vi "GetTaskInfo.vi"(0 "error in":errorcluster, 5 "Telnet":refnum<k24>, 9 "task":string) -> (4 "error out":errorcluster, 6 "KclCommand":string, 8 "Succeed":bool, 10 "ErrorText":string, 15 "TaskInfo":T1)   [LabVIEW 2024, in "UnderAutomation.Fanuc.lvlib"]
uses:
  UnderAutomation.Fanuc.lvlib
  C:/Users/fg/Documents/Fanuc.vi/LabVIEW_2024/UnderAutomation.Fanuc/lib/UnderAutomation.Fanuc.dll
  lib/UnderAutomation.Fanuc.dll
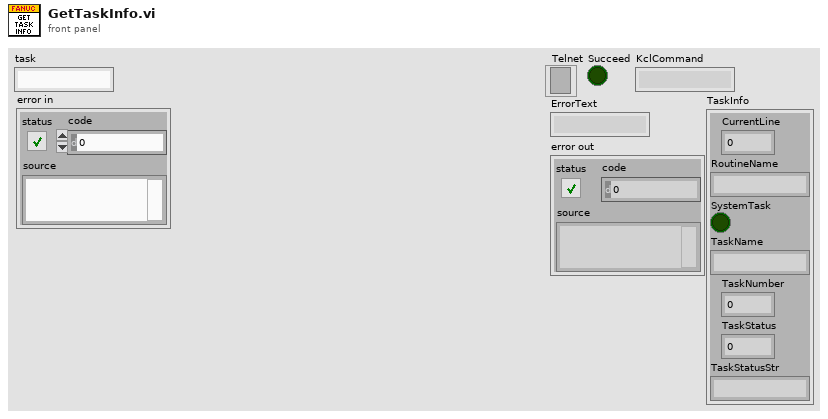
[diagram p1: front panel]
types:
  T1 = cluster{"CurrentLine":i32, "RoutineName":string, "SystemTask":bool, "TaskName":string, "TaskNumber":i32, "TaskStatus":i32, "TaskStatusStr":string}
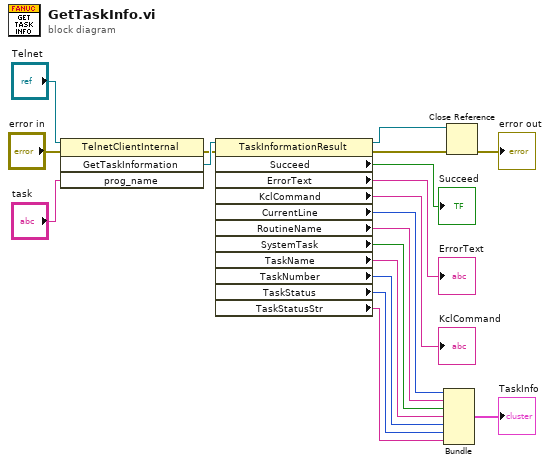
[diagram p0: block diagram]
diagram:
  n1 = invoke class="TelnetClientInternal" method="GetTaskInformation"(reference="Telnet", error in="error in", "prog_name"="task") -> (error out=w14:errorcluster, "GetTaskInformation"=w17:refnum<k24>)  [unwired: 1 in, 2 out]
  n2 = property class="TaskInformationResult"(reference=w17, error in=w14) -> (reference out=w10:refnum<k24>, error out=w11:errorcluster, "Succeed"=→"Succeed":bool, "ErrorText"=→"ErrorText":string, "KclCommand"=→"KclCommand":string, "CurrentLine"=w8:i32, "RoutineName"=w7:string, "SystemTask"=w6:bool, "TaskName"=w5:string, "TaskNumber"=w4:i32, "TaskStatus"=w3:i32, "TaskStatusStr"=w2:string)
  n3 = Bundle("CurrentLine"=w8, "RoutineName"=w7, "SystemTask"=w6, "TaskName"=w5, "TaskNumber"=w4, "TaskStatus"=w3, "TaskStatusStr"=w2) -> (→"TaskInfo":T1)  [unwired: 1 in]
  n4 = Close Reference(reference=w10, error in (no error)=w11) -> (error out=→"error out":errorcluster)
